vi "theta1.vi"(8 "L1":i32, 9 "l0":i32, 10 "Numeric 2":dbl, 11 "Numeric":dbl) -> (3 "Numeric 5":dbl)   [LabVIEW 2014]
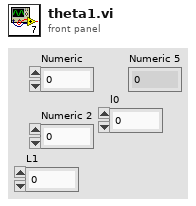
[diagram p1: front panel]
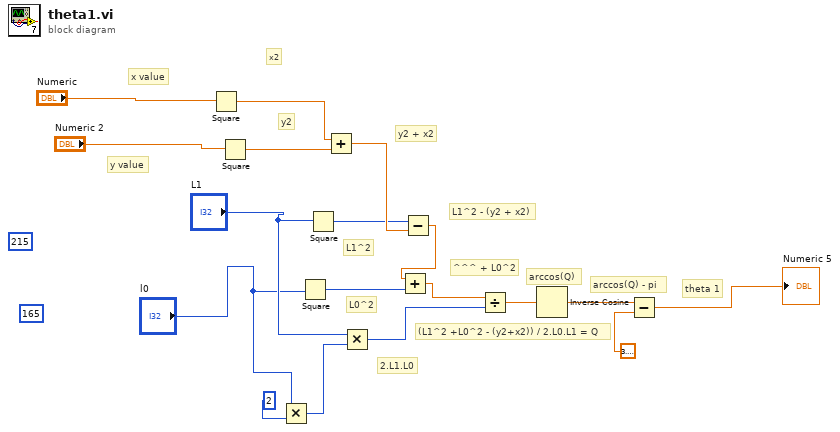
[diagram p0: block diagram]
diagram:
  (unwired) 165
  (unwired) 215
  # "y value"
  # "x value"
  # "theta 1"
  # "arccos(Q) - pi"
  # "arccos(Q)"
  # "(L1^2 +L0^2 - (y2+x2)) / 2.L0.L1 = Q"
  # "2.L1.L0"
  # "^^^ + L0^2"
  # "L1^2 - (y2 + x2)"
  # "L0^2"
  # "L1^2"
  # "y2 + x2"
  # "x2"
  # "y2"
  n1 = Square(x="Numeric") -> (x^2=w18:dbl)
  n2 = Square(x="Numeric 2") -> (x^2=w17:dbl)
  n3 = Multiply(x="l0", y=2) -> (x*y=w11:i32)
  n4 = Square(x="l0") -> (x^2=w14:i32)
  n5 = Square(x="L1") -> (x^2=w15:i32)
  n6 = Add(x=w18, y=w17) -> (x+y=w16:dbl)
  n7 = Multiply(x="L1", y=w11) -> (x*y=w9:i32)
  n8 = Subtract(x=w15, y=w16) -> (x-y=w13:dbl)
  n9 = Add(x=w13, y=w14) -> (x+y=w12:dbl)
  n10 = Divide(x=w12, y=w9) -> (x/y=w8:dbl)
  n11 = Inverse Cosine(1:w8) -> (0:w7:dbl)
  n12 = Subtract(x=w7, y=3.141592653589793) -> (x-y=→"Numeric 5":dbl)
